vi "Blue_Green.vi"() -> (3 "Refnum out":T1)   [LabVIEW 2018]
uses:
  <vilib>/vision/Image Controls.llb/IMAQ Image.ctl
panel:
  in  "File Path 2":path=path "D:/Life/20191001_Accordance/Project/EPISIL/20200806-Camera/20200716/getimg_003.bmp"
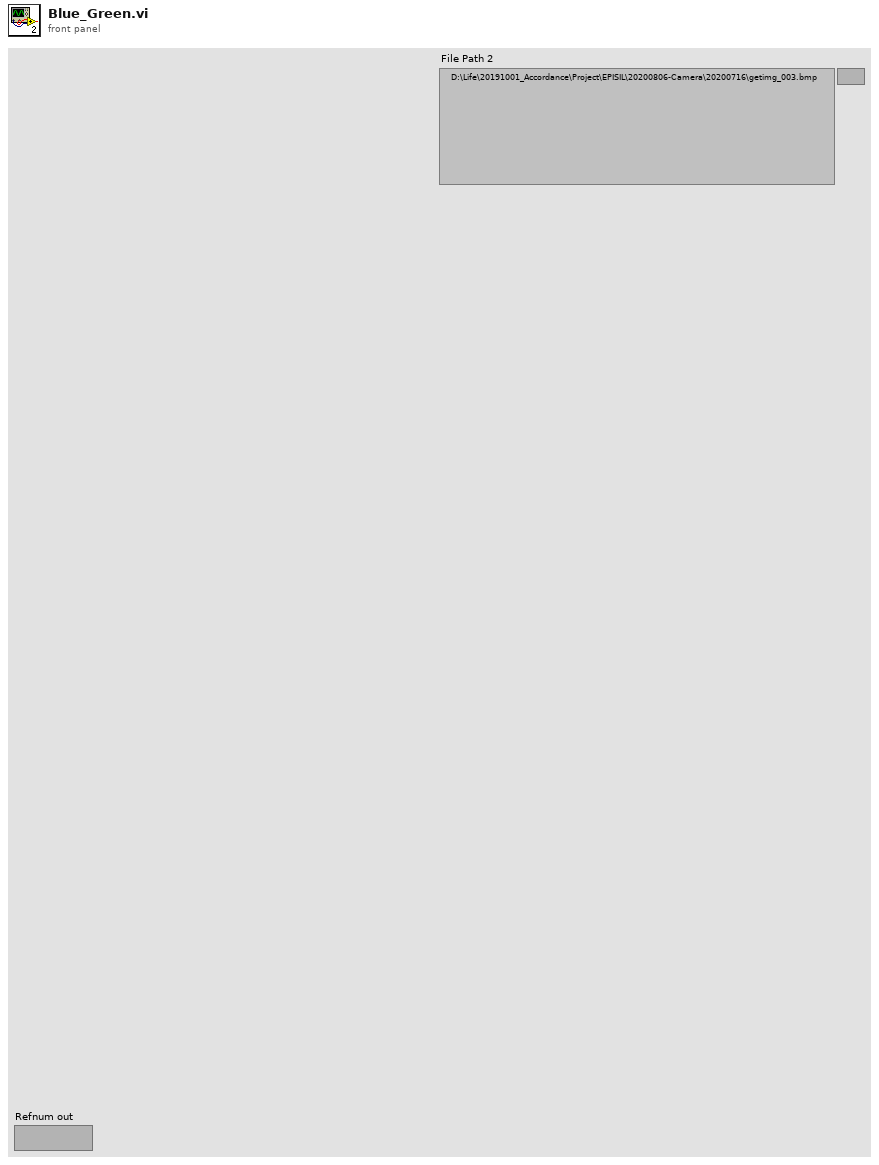
[diagram p1: front panel]
types:
  T1 = typedef "IMAQ Image.ctl" = refnum<image>
  T2 = typedef "Image Type" = u32
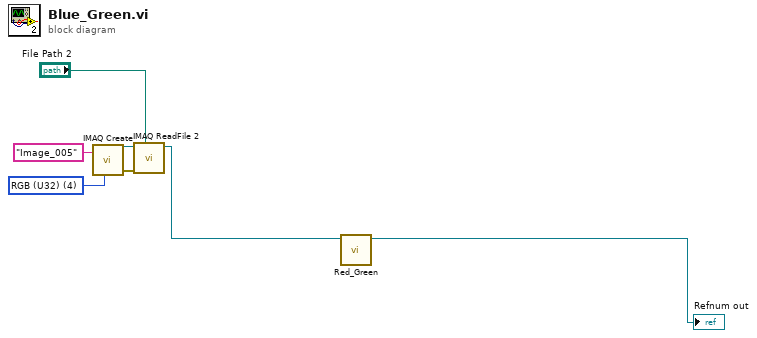
[diagram p0: block diagram]
diagram:
  w3 = T2 4 items=["Grayscale (U8)", "Grayscale (I16)", "Grayscale (SGL)", "Complex (CSG)", "RGB (U32)", "HSL (U32)", "RGB (U64)", "Grayscale (U16)"] ("Image Type")
  n1 = call "IMAQ Create"("Image Name"="Image_005", "Image Type"=w3) -> ("New Image"=w4:T1, "error out"=w5:errorcluster)  [unwired: 3 in]
  n2 = call "IMAQ ReadFile 2"("File Path"="File Path 2", "error in (no error)"=w5, "Image"=w4) -> ("Image Out"=w1:T1)  [unwired: 4 in, 4 out]
  n3 = call "Red_Green.vi"("Refnum in"=w1) -> ("Refnum out"=→"Refnum out":T1)  [unwired: 9 in, 1 out]
